vi "RX Disabled channel logic 4ch 4SPC.vi"(7 "reset":bool, 9 "input valid":bool, 10 "data":u32[](array[numeric])=[0, 0, 0, 0, 0, 0, 0, 0, 0, 0, 0, 0, 0, 0, 0, 0], 11 "enabled channels":u32) -> (1 "data ready":bool, 2 "data out":u32[](array[numeric]))   [LabVIEW 2025, in "niUSRP Stream Control (DMA) v1 FPGA.lvclass"]
uses:
  niUSRP Stream Control (DMA) v1 FPGA.lvclass
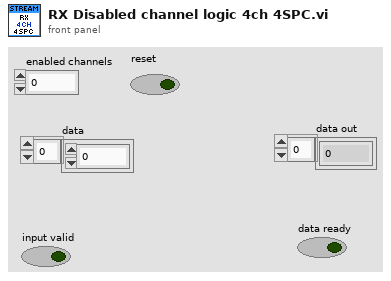
[diagram p1: front panel]
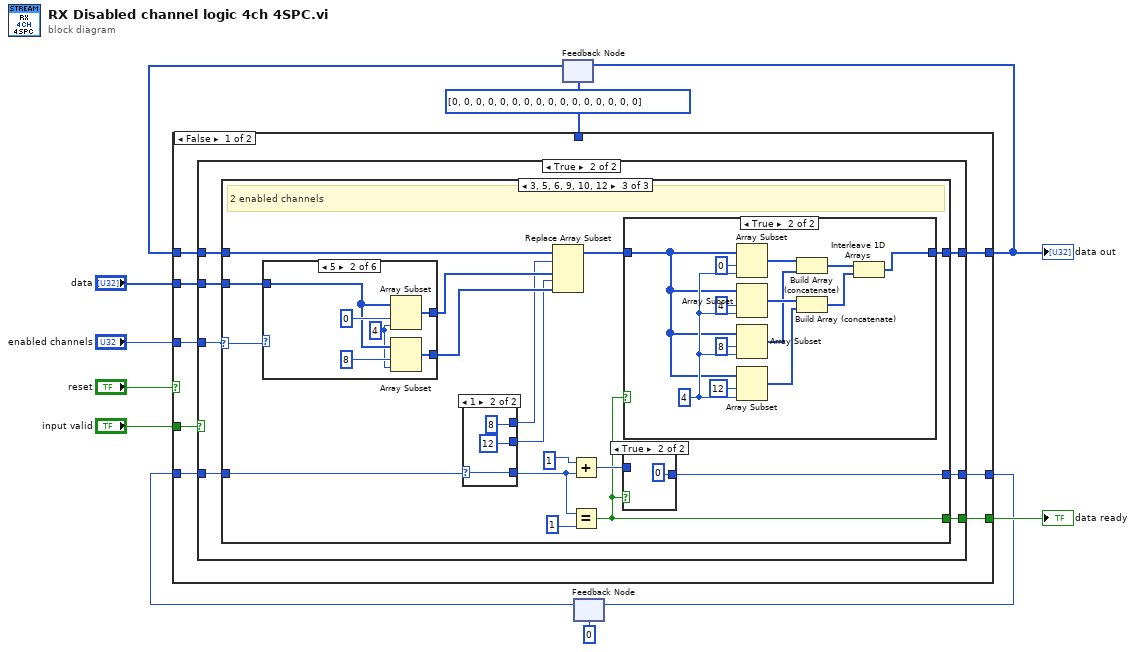
[diagram p0: block diagram]
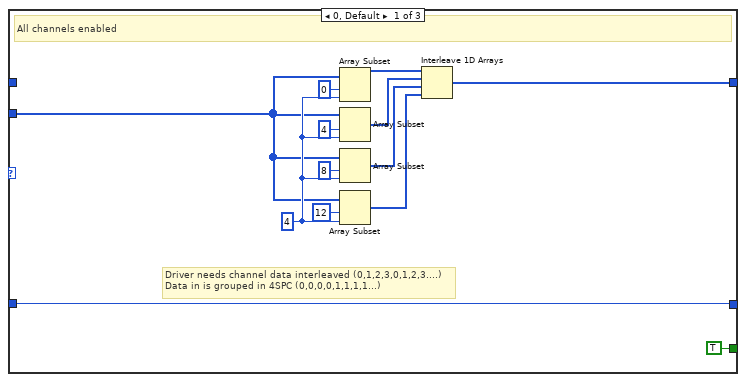
[diagram p3: hidden frame]
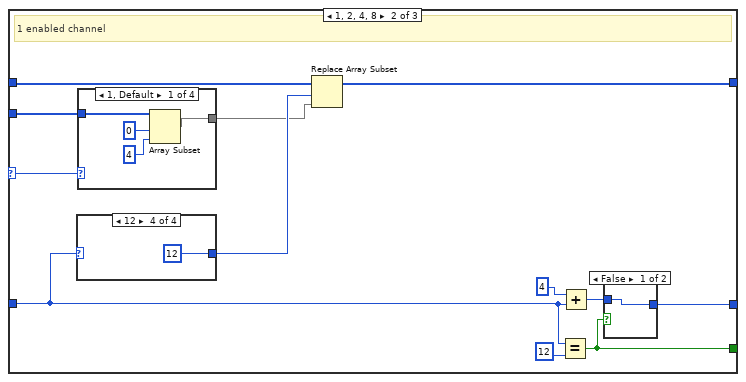
[diagram p4: hidden frame]
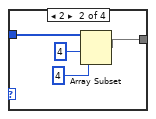
[diagram p5: hidden frame]
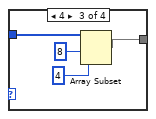
[diagram p6: hidden frame]
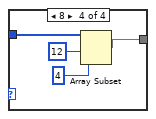
[diagram p7: hidden frame]
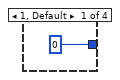
[diagram p8: hidden frame]
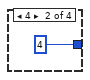
[diagram p9: hidden frame]
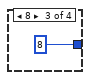
[diagram p10: hidden frame]
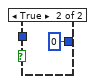
[diagram p11: hidden frame]
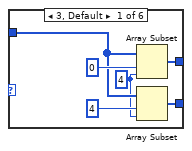
[diagram p13: hidden frame]
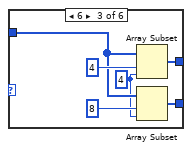
[diagram p14: hidden frame]
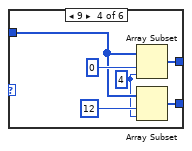
[diagram p15: hidden frame]
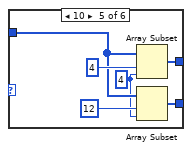
[diagram p16: hidden frame]
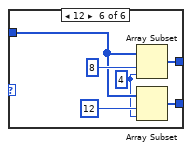
[diagram p17: hidden frame]
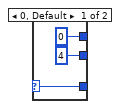
[diagram p18: hidden frame]
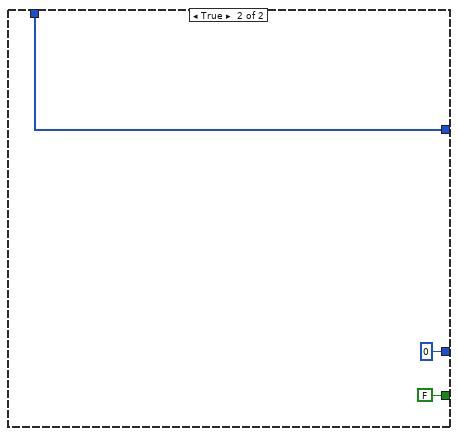
[diagram p20: hidden frame]
diagram:
  w1 = u32[] [0, 0, 0, 0, 0, 0, 0, 0, 0, 0, 0, 0, 0, 0, 0, 0]
  n1 = feedback #1(w1) -> (w11:u32[])
  n2 = feedback #2(u8 0) -> (w4:u8)
  n3 = case shown="False" "reset" {
    tunnel: w11 -> [w19 _]
    tunnel: "enabled channels" -> [w18 _]
    tunnel: "data" -> [w17 _]
    tunnel: [w16 FALSE] -> w8
    tunnel: "input valid" -> [w15 _]
    tunnel: [w14 u8 0] -> w5
    tunnel: w4 -> [w13 _]
    tunnel: [w12 w151] -> w3
    tunnel: w1 -> [_ w151]
    frame False {
      n4 = case shown="True" w15 {
        selector: w15 -> [w20 _]
        tunnel: [w22 w23] -> w12
        tunnel: w19 -> [w22 w29]
        tunnel: w17 -> [_ w28]
        tunnel: w18 -> [_ w27]
        tunnel: [w21 w25] -> w14
        tunnel: w13 -> [w21 w26]
        tunnel: [w20 w24] -> w16
        frame False {
        }
        frame True {
          n5 = case shown="3, 5, 6, 9, 10, 12" w27 {
            selector: w27 -> [_ w46 w80]
            tunnel: w28 -> [w30 w45 w88]
            tunnel: [w31 w53 w77] -> w23
            tunnel: [TRUE w51 w79] -> w24
            tunnel: w26 -> [w42 w48 w84]
            tunnel: [w42 w49 w89] -> w25
            tunnel: w29 -> [_ w52 w91]
            frame 0, Default {
              w40 = 4 ("length")
              # "Driver needs channel data interleaved (0,1,2,3,0,1,2,3....)\nData in is grouped in 4SPC (0,0,0,0,1,1,1,1...)"
              # "All channels enabled"
              n6 = Array Subset(array=w30, index=0, length=w40) -> (w35:u32[])
              n7 = Array Subset(array=w30, index=4, length=w40) -> (w34:u32[])
              n8 = Array Subset(array=w30, index=8, length=w40) -> (w33:u32[])
              n9 = Array Subset(array=w30, index=12, length=w40) -> (w32:u32[])
              n10 = Interleave 1D Arrays(w35, w34, w33, w32) -> (w31:u32[])
            }
            frame 1, 2, 4, 8 {
              # "1 enabled channel"
              n11 = case shown="12" w48 {
                tunnel: [0 ("index") 4 ("index") 8 ("index") 12 ("index")] -> w47
                frame 1, Default {
                }
                frame 4 {
                }
                frame 8 {
                }
                frame 12 {
                }
              }
              n12 = case shown="1, Default" w46 {
                tunnel: [w55 w59 w63 w67] -> w44
                tunnel: w45 -> [w58 w62 w66 w70]
                frame 1, Default {
                  n13 = Array Subset(array=w58, index=0, length=4) -> (w55:u32[])
                }
                frame 2 {
                  n14 = Array Subset(array=w62, index=4, length=4) -> (w59:u32[])
                }
                frame 4 {
                  n15 = Array Subset(array=w66, index=8, length=4) -> (w63:u32[])
                }
                frame 8 {
                  n16 = Array Subset(array=w70, index=12, length=4) -> (w67:u32[])
                }
              }
              n17 = Replace Array Subset(array=w52, new element=w44, index=w47) -> (w53:u32[])
              n18 = Equal?(x=w48, y=u8 12) -> (x = y?=w51:bool)
              n19 = Add(x=u8 4 ("length"), y=w48) -> (x+y=w50:u8)
              n20 = case shown="False" w51 {
                tunnel: [w75 u8 0] -> w49
                tunnel: w50 -> [w75 _]
                frame False {
                }
                frame True {
                }
              }
            }
            frame 3, 5, 6, 9, 10, 12 {
              # "2 enabled channels"
              n21 = case shown="5" w80 {
                tunnel: w88 -> [w111 w117 w123 w129 w135 w141]
                tunnel: [w109 w115 w121 w127 w133 w139] -> w87
                tunnel: [w108 w114 w120 w126 w132 w138] -> w86
                frame 3, Default {
                  w107 = 4 ("length")
                  n22 = Array Subset(array=w111, index=0, length=w107) -> (w109:u32[])
                  n23 = Array Subset(array=w111, index=4, length=w107) -> (w108:u32[])
                }
                frame 5 {
                  w113 = 4 ("length")
                  n24 = Array Subset(array=w117, index=0, length=w113) -> (w115:u32[])
                  n25 = Array Subset(array=w117, index=8, length=w113) -> (w114:u32[])
                }
                frame 6 {
                  w119 = 4 ("length")
                  n26 = Array Subset(array=w123, index=4, length=w119) -> (w121:u32[])
                  n27 = Array Subset(array=w123, index=8, length=w119) -> (w120:u32[])
                }
                frame 9 {
                  w125 = 4 ("length")
                  n28 = Array Subset(array=w129, index=0, length=w125) -> (w127:u32[])
                  n29 = Array Subset(array=w129, index=12, length=w125) -> (w126:u32[])
                }
                frame 10 {
                  w131 = 4 ("length")
                  n30 = Array Subset(array=w135, index=4, length=w131) -> (w133:u32[])
                  n31 = Array Subset(array=w135, index=12, length=w131) -> (w132:u32[])
                }
                frame 12 {
                  w137 = 4 ("length")
                  n32 = Array Subset(array=w141, index=8, length=w137) -> (w139:u32[])
                  n33 = Array Subset(array=w141, index=12, length=w137) -> (w138:u32[])
                }
              }
              n34 = case shown="1" w84 {
                selector: w84 -> [w145 w148]
                tunnel: [w145 w148] -> w83
                tunnel: [0 ("index") 8 ("index")] -> w82
                tunnel: [4 ("index") 12 ("index")] -> w81
                frame 0, Default {
                }
                frame 1 {
                }
              }
              n35 = Replace Array Subset(array=w91, new element #1=w87, index #1=w82, new element #2=w86, index #2=w81) -> (w78:u32[])
              n36 = Add(x=u8 1, y=w83) -> (x+y=w90:u8)
              n37 = Equal?(x=w83, y=u8 1) -> (x = y?=w79:bool)
              n38 = case shown="True" w79 {
                tunnel: [w149 u8 0] -> w89
                tunnel: w90 -> [w149 _]
                frame False {
                }
                frame True {
                }
              }
              n39 = case shown="True" w79 {
                tunnel: [w93 w100] -> w77
                tunnel: w78 -> [w93 w101]
                frame False {
                }
                frame True {
                  w106 = 4 ("length")
                  n40 = Array Subset(array=w101, index=0, length=w106) -> (w99:u32[])
                  n41 = Array Subset(array=w101, index=4, length=w106) -> (w98:u32[])
                  n42 = Array Subset(array=w101, index=8, length=w106) -> (w97:u32[])
                  n43 = Array Subset(array=w101, index=12, length=w106) -> (w96:u32[])
                  n44 = Build Array (concatenate)(w99, w97) -> (w95:u32[])
                  n45 = Build Array (concatenate)(w98, w96) -> (w94:u32[])
                  n46 = Interleave 1D Arrays(w95, w94) -> (w100:u32[])
                }
              }
            }
          }
        }
      }
    }
    frame True {
    }
  }
  "data out" <- w3
  "data ready" <- w8
  n47 = feedback-in #1(w3) -> ()
  n48 = feedback-in #2(w5) -> ()
